vi "Write Redirect URI.vi"(8 "error in (no error)":errorcluster, 10 "Redirect URI":string="http://localhost:58888/Oauth2/Redirect", 11 "Oauth2 in":refnum<class "Oauth2.lvclass">) -> (0 "error out":errorcluster, 3 "Oauth2 out":refnum<class "Oauth2.lvclass">)   [LabVIEW 2020, in "Oauth2.lvclass"]
uses:
  Oauth2.lvclass
  Oauth2.lvclass/Oauth2.ctl
  <vilib>/LabVIEW Open Source Project/OpenURI/uri/URI.lvclass
  OAuthToken/OAuthAccessToken.lvclass
  OAuthToken/OAuth2 Token Element -- enum.ctl
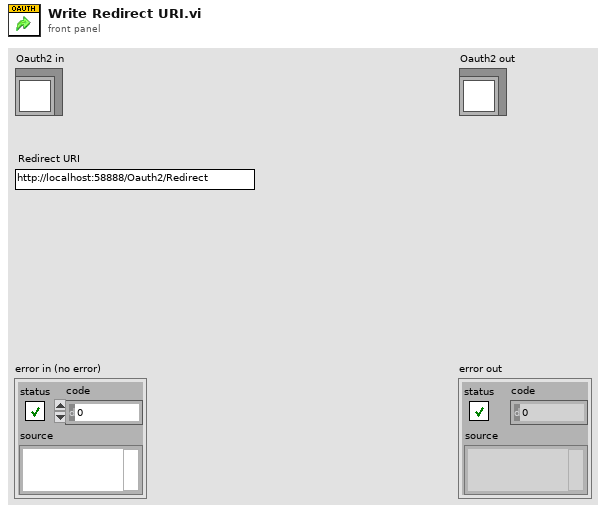
[diagram p1: front panel]
types:
  T1 = typedef "OAuthAccessToken.lvclass/OAuth2 Token Element -- enum.ctl" = enum16{"client_id", "client_secret", "response_type", "scope", "redirect_uri", "error", "error_description", "error_uri", "grant_type", "code", "access_token", "token_type", "expires_in", "username", "password", "refresh_token", "code_challenge", "code_challenge_method", "reverse_proxy_uri", "endpoint element"}
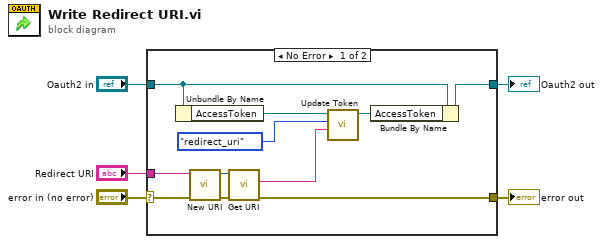
[diagram p0: block diagram]
diagram:
  n1 = case shown="No Error" "error in (no error)" {
    selector: "error in (no error)" -> [w7 w17]
    tunnel: [w6 w17] -> w4
    tunnel: [w9 w18] -> w2
    tunnel: "Oauth2 in" -> [w12 w18]
    tunnel: "Redirect URI" -> [w16 _]
    frame No Error {
      n2 = Unbundle By Name(w12) -> ("AccessToken"=w14:refnum<class "OAuthAccessToken.lvclass">)
      n3 = call <vilib>:"New URI.vi"("error in (no error)"=w7, "URI"=w16) -> ("error out"=w8:errorcluster, "URI"=w11:refnum<class "URI.lvclass">)  [unwired: 8 in]
      n4 = call <vilib>:"Get URI.vi"("error in (no error)"=w8, "URI in"=w11) -> ("error out"=w6:errorcluster, "URI String"=w10:string)  [unwired: 7 in, 1 out]
      n5 = call "Update Token.vi"("Value"=w10, "Token element"=OAuth2_Token_Element_--_enum."redirect_uri", "OAuthAccessToken in"=w14) -> ("OAuthAccessToken out"=w15:refnum<class "OAuthAccessToken.lvclass">)  [unwired: 7 in, 1 out]
      n6 = Bundle By Name(cluster=w12, "AccessToken"=w15) -> (w9:refnum<class "Oauth2.lvclass">)
    }
    frame Error {
    }
  }
  "error out" <- w4
  "Oauth2 out" <- w2
